vi "XDataNode_OnFontChange.vi"(0 "XRef":refnum<vi>, 1 "State In":T1 {"Timing"."I/O Scan Engine Mode" max=255 format="%#.0f"; "Timing"."Assigned CPU" min=-2 max=255 format="%#.0f"}) -> (14 "Reply":string[](array[string]), 15 "State Out":T1 {"Timing"."I/O Scan Engine Mode" max=255 format="%#.0f"; "Timing"."Assigned CPU" min=-2 max=255 format="%#.0f"})   [LabVIEW 2017, in "XDataNode.xnode"]
uses:
  XDataNode.xnode
panel:
  # "Expected End [f-1]"
  # "Actual End [f-1]"
  # "Finished Late? [f-1]"
  # "Expected End [i-1]"
  # "Actual End [i-1]"
  # "Finished Late? [i-1]"
  # "Exp.Iter.Start"
  # "Act.Iter.Start"
  # "Exp.Frm.Start"
  # "Act.Frm.Start"
  # "Source Name"
  # "Loop/Sequence Name"
  # "Period"
  # "Deadline"
  # "Offset"
  # "Start"
  # "Priority"
  # "Timeout"
  # "Mode"
  # "Wakeup Reason"
  # "Error"
  # "Source Type"
  # "2nd.Src.Type"
  # "Global End Time"
  # "Global Start Time"
  # "Frame Duration"
  # "Iteration Duration"
  # "Assigned CPU"
  # "I/O Scan Engine Mode"
  # "Expected End [f-1]"
  # "Actual End [f-1]"
  # "Finished Late? [f-1]"
  # "Expected End [i-1]"
  # "Actual End [i-1]"
  # "Finished Late? [i-1]"
  # "Exp.Iter.Start"
  # "Act.Iter.Start"
  # "Exp.Frm.Start"
  # "Act.Frm.Start"
  # "Source Name"
  # "Loop/Sequence Name"
  # "Period"
  # "Deadline"
  # "Offset"
  # "Start"
  # "Priority"
  # "Timeout"
  # "Mode"
  # "Wakeup Reason"
  # "Error"
  # "Source Type"
  # "2nd.Src.Type"
  # "Global End Time"
  # "Global Start Time"
  # "Frame Duration"
  # "Iteration Duration"
  # "Assigned CPU"
  # "I/O Scan Engine Mode"
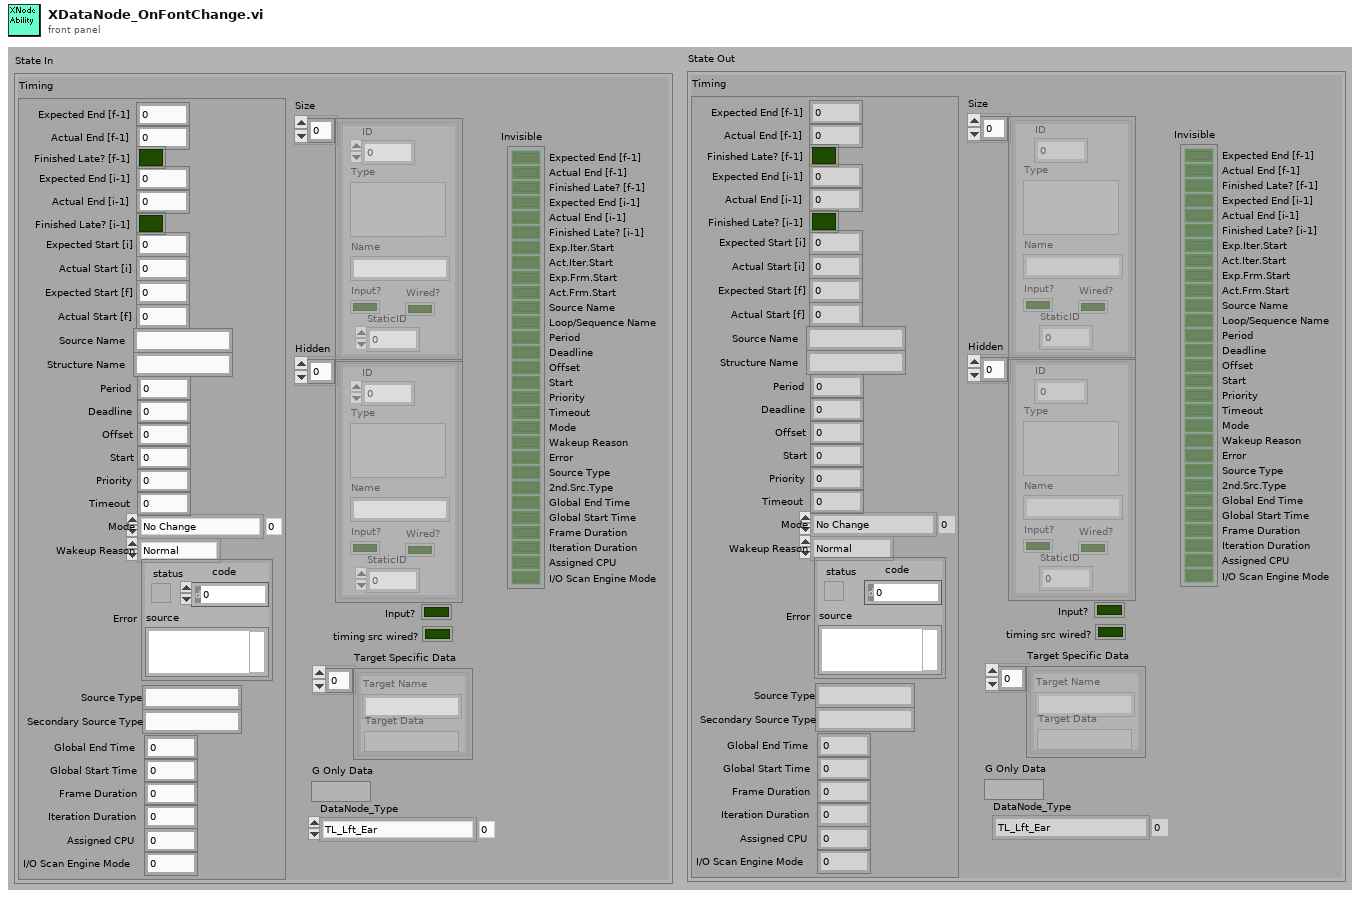
[diagram p1: front panel]
types:
  T1 = cluster{"Timing":cluster{"Expected End [f-1]":u64, "Actual End [f-1]":u64, "Finished Late? [f-1]":bool, "Expected End [i-1]":u64, "Actual End [i-1]":u64, "Finished Late? [i-1]":bool, "Expected Start [i]":u64, "Actual Start [i]":u64, "Expected Start [f]":u64, "Actual Start [f]":u64, "Source Name":string, "Structure Name":string, "Period":i64, "Deadline":i64, "Offset":i64, "Start":i64, "Priority":i32, "Timeout":i32, "Mode":enum32{"No Change", "Process missed periods, maintain original phase", "Discard missed periods, maintain original phase", "Process missed periods, ignore original phase", "Discard missed periods, ignore original phase"}, "Wakeup Reason":enum32{"Normal", "Aborted", "Asynchronous wakeup", "Timing source error", "Timed loop error", "Timeout"}, "Error":errorcluster, "Source Type":string, "Secondary Source Type":string, "Global End Time":u64, "Global Start Time":u64, "Frame Duration":u64, "Iteration Duration":u64, "Assigned CPU":i32, "I/O Scan Engine Mode":u32}, "Size":cluster{"ID":i32, "Wired?":bool, "Type":variant, "Name":string, "Input?":bool, "StaticID":i32}[], "Hidden":cluster{"ID":i32, "Wired?":bool, "Type":variant, "Name":string, "Input?":bool, "StaticID":i32}[], "Invisible":bool[], "Input?":bool, "timing src wired?":bool, "Target Specific Data":cluster{"Target Name":string, "Target Data":variant}[], "G Only Data":variant, "DataNode_Type":enum32{"TL_Lft_Ear", "TL_Rt_Ear", "TL_Lft_Dn", "TL_Rt_Dn", "TS_Lft_Ear", "TS_Rt_Ear", "TS_1stFrame_Lft_Dn", "TS_Lft_Dn", "TS_LastFrame_Rt_Dn", "TS_Rt_Dn", "TL_TS_Lft_Ear", "TL_TS_Rt_Ear", "TL_TS_Lft_Dn", "TL_TS_Rt_Dn", "TL_TS_1stFrame_Lft_Dn", "TL_TS_LastFrame_Rt_Dn"}}
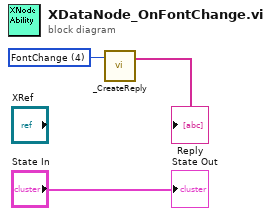
[diagram p0: block diagram]
diagram:
  w1 = u16 4 items=["FullUpdate", "RefeeChanged", "AdaptToInputs", "Refresh", "FontChange"] ("Ring")
  n1 = call "_CreateReply.vi"("Ring"=w1) -> ("Reply"=→"Reply":string[])  [unwired: 2 in]
  "State Out" <- "State In"
